vi "ReadFile.vi"(8 "error in (no error)":errorcluster, 11 "File in":refnum<class "File.lvclass">) -> (0 "error out":errorcluster, 2 "data":i32[](array[numeric]))   [LabVIEW 2021, in "File.lvclass"]
uses:
  File.lvclass
  File.lvclass/File.ctl
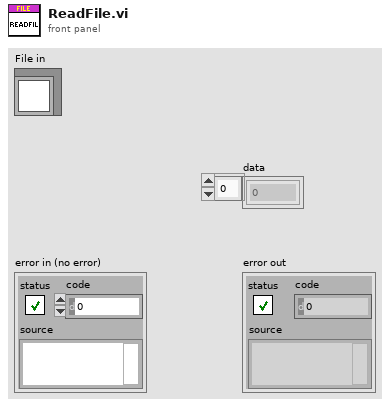
[diagram p1: front panel]
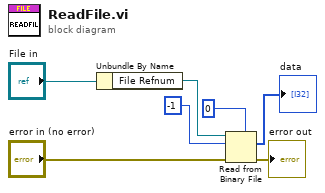
[diagram p0: block diagram]
diagram:
  n1 = Unbundle By Name("File in") -> ("File Refnum"=w3:refnum<file>)
  n2 = Read from Binary File(5:0, 8:"error in (no error)", 10:-1 ("count (1)"), 11:w3) -> (0:→"error out":errorcluster, 2:→"data":i32[])  [unwired: 2 in, 2 out]
